vi "handleMsgDetails.vi"(8 "error in (no error)":errorcluster, 10 "msgTypeDef in":T1={"msgName"="move", "msgDetails"="\"tolerance\":2,"}, 11 "TcpServer.lvclass":refnum<class "TcpServer.lvclass">) -> (0 "error out":errorcluster, 2 "msgTypeDef out":T1={"msgName"="move", "msgDetails"="\"tolerance\":2,"}, 3 "TcpServer.lvclass":refnum<class "TcpServer.lvclass">)   [LabVIEW 2018, in "TcpServer.lvclass"]
doc: "Read every line with message details, remove empty lines and add a comma to them. This new string will be converted into JSON string in formatMsgDetails.vi."
uses:
  TcpServer.lvclass
  typedef/msgTypeDef.ctl
  <vilib>/regexp/Match Regular Expression.xnode
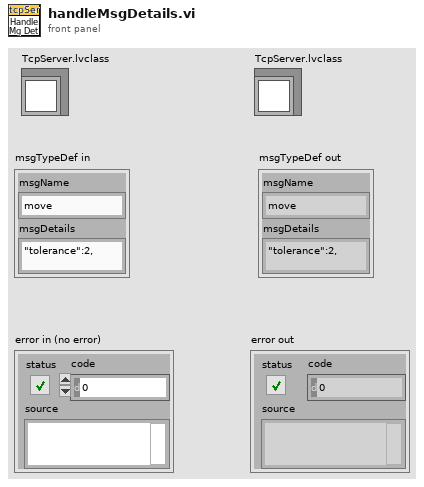
[diagram p1: front panel]
types:
  T1 = typedef "TcpServer.lvclass/msgTypeDef.ctl" = cluster{"msgName":string, "msgDetails":string}
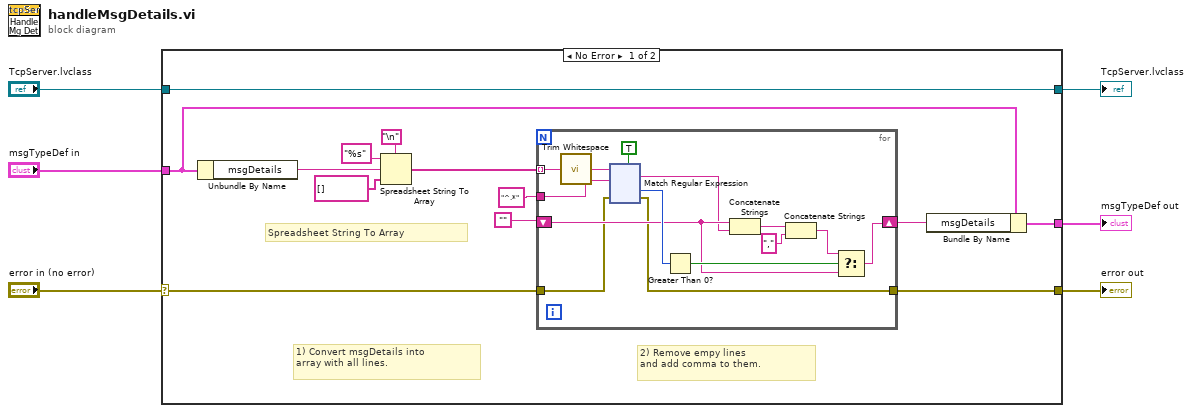
[diagram p0: block diagram]
diagram:
  n1 = case shown="No Error" "error in (no error)" {
    selector: "error in (no error)" -> [w13 w149]
    tunnel: [w12 w149] -> w5
    tunnel: "TcpServer.lvclass" -> [w11 w150]
    tunnel: [w11 w150] -> w3
    tunnel: "msgTypeDef in" -> [w8 w148]
    tunnel: [w7 w148] -> w1
    frame No Error {
      # "Spreadsheet String To Array"
      # "2) Remove empy lines\nand add comma to them."
      # "1) Convert msgDetails into\narray with all lines."
      n2 = Unbundle By Name(w8) -> ("msgDetails"=w10:string)
      n3 = Spreadsheet String To Array(delimiter (Tab)="\n", format string="%s", spreadsheet string=w10, array type (2D Dbl)=string[] [] ("format string")) -> (array=w14:string[])
      n4 = for {
        tunnel: w14 -> [w30] mode=indexing
        tunnel: "^.*" -> [w33]
        shift-right: [w27] -> w9
        shift-left: "" -> [w23]
        tunnel: w13 -> [w21]
        tunnel: [w20] -> w12
        n5 = call <vilib>:"Trim Whitespace.vi"("string"=w30) -> ("trimmed string"=w29:string)  [unwired: 1 in]
        n6 = xnode ("Match Regular Expression")("input string"=w29, "regular expression"=w33, "error in"=w21, "multiline? (F)"=TRUE) -> ("whole match"=w22:string, "offset past match"=w31:i32, "error out"=w20:errorcluster)  [unwired: 2 in, 2 out]
        n7 = Greater Than 0?(x=w31) -> (x > 0?=w28:bool)
        n8 = Concatenate Strings(w23, w22) -> (w26:string)
        n9 = Concatenate Strings(w26, "," ("comma")) -> (w24:string)
        n10 = Select(t=w24, s=w28, f=w23) -> (s? t:f=w27:string)
      }
      n11 = Bundle By Name(cluster=w8, "msgDetails"=w9) -> (w7:T1)
    }
    frame Error {
    }
  }
  "error out" <- w5
  "TcpServer.lvclass" <- w3
  "msgTypeDef out" <- w1
